vi "Remove Known.vi"(8 "error in (no error)":errorcluster, 10 "filenames":string[](array[string]), 11 "Working Dir":path) -> (0 "error out":errorcluster, 1 "Known Found?":bool, 2 "Filenames Out":string[](array[string]), 3 "Working Dir Out":path, 4 "Tags Removed":string[](array[string]))   [LabVIEW 2024]
uses:
  TypeDefs/Tag Cmd.ctl
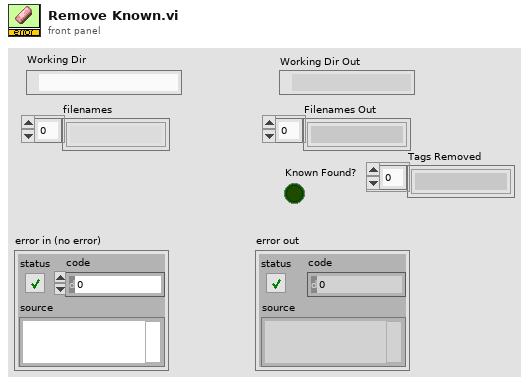
[diagram p1: front panel]
types:
  T1 = typedef "Tag Cmd.ctl" = enum16{"Init", "Get Known", "Set Known"}
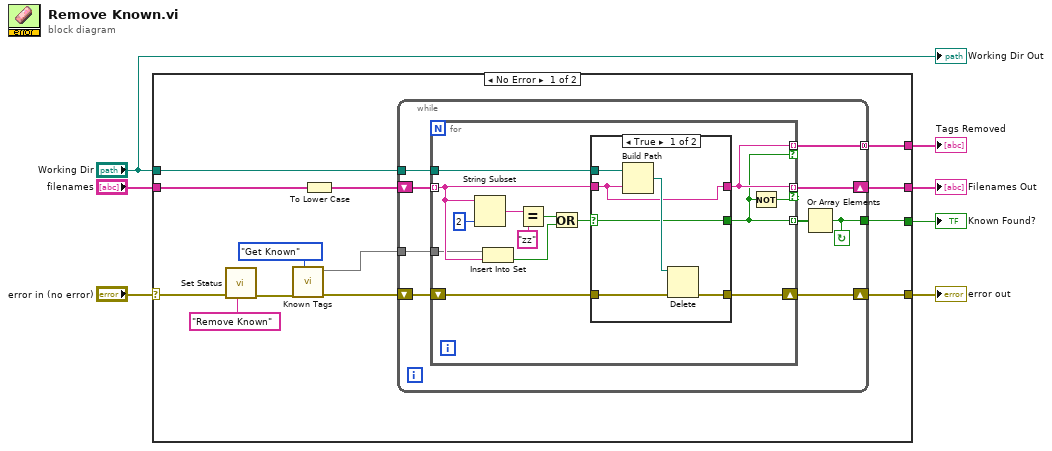
[diagram p0: block diagram]
diagram:
  n1 = case shown="No Error" "error in (no error)" {
    selector: "error in (no error)" -> [w12 w52]
    tunnel: "filenames" -> [w18 _]
    tunnel: [w17 w52] -> w6
    tunnel: "Working Dir" -> [w16 _]
    tunnel: [w15 _] -> w4
    tunnel: [w14 _] -> w3
    tunnel: [w13 _] -> w2
    frame No Error {
      n2 = call "Set Status.vi"("Status Message"="Remove Known" ("Value"), "error in (no error)"=w12) -> ("error out"=w11:errorcluster)  [unwired: 9 in]
      n3 = call "Known Tags.vi"("Tag Cmd"=Tag_Cmd."Get Known", "error in (no error)"=w11) -> ("error out"=w19:errorcluster, "Tag Set"=w9:set{string})  [unwired: 8 in]
      n4 = To Lower Case(string=w18) -> (all lower case string=w8:string[])
      n5 = while {
        tunnel: w9 -> [w27]
        tunnel: w16 -> [w25]
        tunnel: [w22] -> w14
        shift-right: [w26] -> w17
        shift-left: w19 -> [w29]
        shift-right: [w23] -> w15
        shift-left: w8 -> [w28]
        tunnel: [w21] -> w13 mode=concatenating
        stop <- w22 continue-if-true
        n6 = for {
          shift-right: [w42] -> w26
          shift-left: w29 -> [w43]
          tunnel: w28 -> [w40] mode=indexing
          tunnel: w27 -> [w31]
          tunnel: w25 -> [w41]
          tunnel: [w37] -> w24 mode=indexing
          tunnel: [w38] -> w23 mode=indexing if=w39
          tunnel: [w38] -> w21 mode=indexing if=w37
          n7 = String Subset(string=w40, length (rest)=2 ("length (rest)")) -> (substring=w35:string)  [unwired: 1 in]
          n8 = Insert Into Set(10:w40, 11:w31) -> (2:w30:bool)  [unwired: 1 out]
          n9 = Equal?(x=w35, y="zz") -> (x = y?=w32:bool)
          n10 = Or(x=w32, y=w30) -> (x .or. y?=w33:bool)
          n11 = case shown="True" w33 {
            selector: w33 -> [w44 _]
            tunnel: w43 -> [w49 w51]
            tunnel: [w48 w51] -> w42
            tunnel: w41 -> [w47 _]
            tunnel: w40 -> [w45 w50]
            tunnel: [w44 _] -> w37
            tunnel: [w45 w50] -> w38
            frame True {
              n12 = Build Path(base path=w47, name or relative path=w45) -> (appended path=w46:path)
              n13 = Delete(path (use dialog)=w46, error in=w49) -> (error out=w48:errorcluster)  [unwired: 3 in, 2 out]
            }
            frame False {
            }
          }
          n14 = Not(x=w37) -> (.not. x?=w39:bool)
        }
        n15 = Or Array Elements(Boolean array=w24) -> (logical OR=w22:bool)
      }
    }
    frame Error {
    }
  }
  "error out" <- w6
  "Known Found?" <- w3
  "Filenames Out" <- w4
  "Tags Removed" <- w2
  "Working Dir Out" <- "Working Dir"
